vi "Refresh ESTTL Listbox.vi"(5 "AdaptMode":u32, 8 "Setup":T1[](array[typedef]) {"Skip Fire Index" max=7; "Angles"."Duration [s]" format="%#_3p"; "Frequency [Hz]" format="%#_3p"}, 9 "Names":string[](array[string]), 11 "_ESTTL Channels":refnum<vi>) -> ()   [LabVIEW 2016]
uses:
  <vilib>/Powertrain Controls/Device Drivers/DCM/ESTTL/RT/Setup.ctl
  <vilib>/Powertrain Controls/Device Drivers/DCM/ESTTL/FPGA/Mode.ctl
  <vilib>/Powertrain Controls/Device Drivers/DCM/ESTTL/RT/Angle Control.ctl
  <vilib>/Powertrain Controls/Device Drivers/DCM/ESTTL/FPGA/DCM - FPGA - ESTTL.lvlib
  <vilib>/Powertrain Controls/Device Drivers/DCM/ESTTL/RT/DCM - RT - ESTTL.lvlib
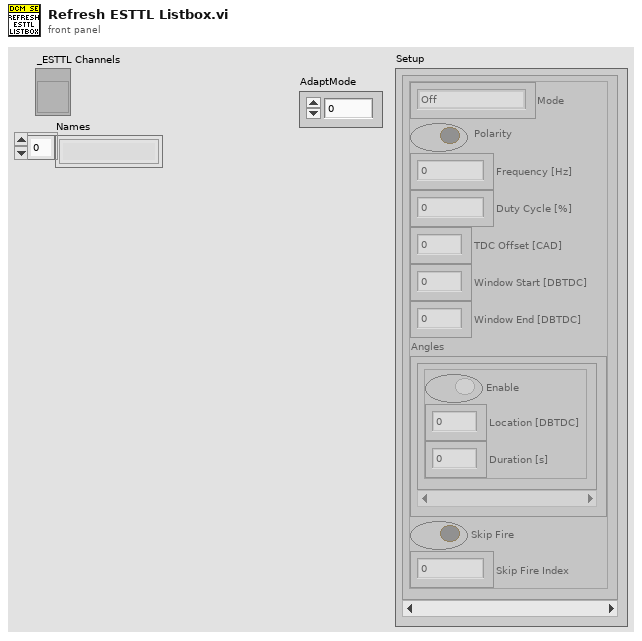
[diagram p1: front panel]
types:
  T1 = typedef "DCM - RT - ESTTL.lvlib/Setup.ctl" = cluster{"Mode":T2, "Polarity":bool, "Frequency [Hz]":sgl, "Duty Cycle [%]":sgl, "TDC Offset [CAD]":sgl, "Window Start [DBTDC]":sgl, "Window End [DBTDC]":sgl, "Angles":T3[], "Skip Fire":bool, "Skip Fire Index":u8}
  T2 = typedef "DCM - FPGA - ESTTL.lvlib/Mode.ctl" = enum8{"Off", "Pulse Width Modulation", "Engine Position Tracking"}
  T3 = typedef "DCM - RT - ESTTL.lvlib/Angle Control.ctl" = cluster{"Enable":bool, "Location [DBTDC]":sgl, "Duration [s]":sgl}
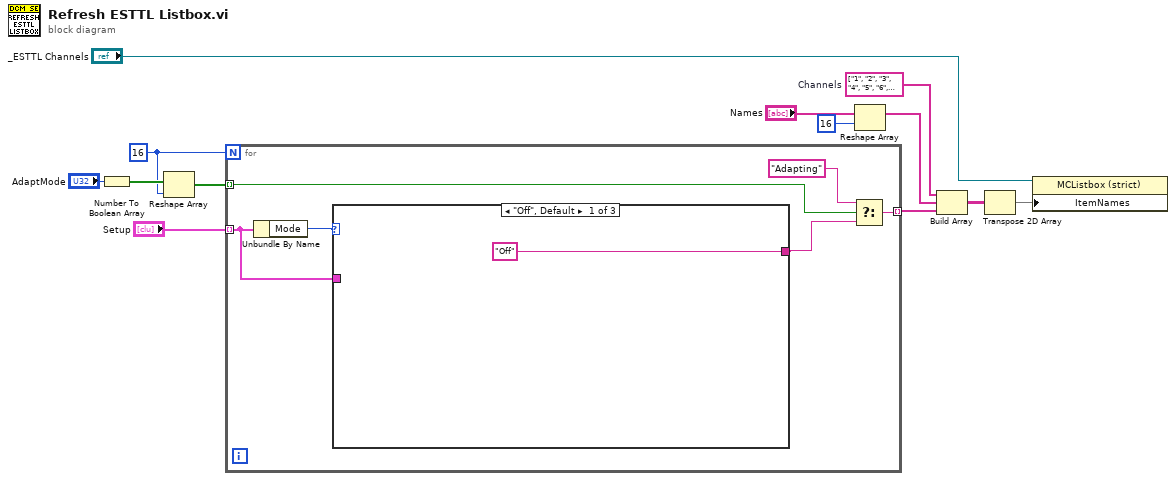
[diagram p0: block diagram]
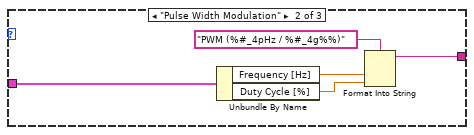
[diagram p2: hidden frame]
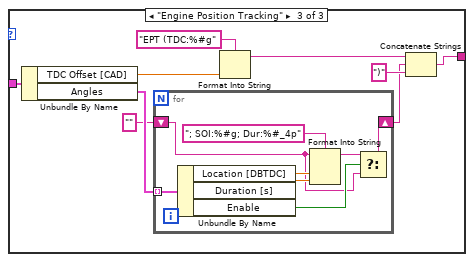
[diagram p3: hidden frame]
diagram:
  w1 = 16
  w11 = string[] ["1", "2", "3", "4", "5", "6", "7", "8", "9", "10", "11", "12", "13", "14", "15", "16"]  # Channels
  n1 = Number To Boolean Array(number="AdaptMode") -> (Boolean array=w5:bool[])
  n2 = Reshape Array(w5, w1) -> (w4:bool[])
  n3 = for {
    N: w1 -> [_]
    tunnel: "Setup" -> [w15] mode=indexing
    tunnel: w4 -> [w18] mode=indexing
    tunnel: [w17] -> w3 mode=indexing
    n4 = Unbundle By Name(w15) -> ("Mode"=w16:T2)
    n5 = case shown="\"Off\", Default" w16 {
      tunnel: w15 -> [_ w25 w33]
      tunnel: ["Off" w21 w29] -> w14
      frame "Off", Default {
      }
      frame "Pulse Width Modulation" {
        n6 = Unbundle By Name(w25) -> ("Frequency [Hz]"=w23:sgl, "Duty Cycle [%]"=w22:sgl)
        n7 = Format Into String(format string="PWM (%#_4pHz / %#_4g%%)", w23, w22) -> (resulting string=w21:string)  [unwired: 2 in, 1 out]
      }
      frame "Engine Position Tracking" {
        n8 = Unbundle By Name(w33) -> ("TDC Offset [CAD]"=w32:sgl, "Angles"=w31:T3[])
        n9 = for {
          tunnel: w31 -> [w40] mode=indexing
          shift-right: [w36] -> w27
          shift-left: "" -> [w35]
          n10 = Unbundle By Name(w40) -> ("Location [DBTDC]"=w41:sgl, "Duration [s]"=w39:sgl, "Enable"=w38:bool)
          n11 = Format Into String(format string="; SOI:%#g; Dur:%#_4p", initial string=w35, w41, w39) -> (resulting string=w37:string)  [unwired: 1 in, 1 out]
          n12 = Select(t=w37, s=w38, f=w35) -> (s? t:f=w36:string)
        }
        n13 = Format Into String(format string="EPT (TDC:%#g", w32) -> (resulting string=w30:string)  [unwired: 2 in, 1 out]
        n14 = Concatenate Strings(w30, w27, ")" ("string")) -> (w29:string)
      }
    }
    n15 = Select(t="Adapting" ("format string"), s=w18, f=w14) -> (s? t:f=w17:string)
  }
  n16 = Reshape Array("Names", 16 ("dimension size")) -> (w8:string[])
  n17 = Build Array(w11, w8, w3) -> (w13:string[][])
  n18 = Transpose 2D Array(2D array=w13) -> (transposed array=w10:string[][])
  n19 = property on="Property Node" class="MCListbox (strict)"(reference="_ESTTL Channels", "ItemNames"=w10) -> ()  [unwired: 1 in, 2 out]
